vi "Get RT Driver Info - 331.vi"(8 "error in (no error)":errorcluster) -> (0 "error out":errorcluster, 1 "RT Driver Info":T1[](array[typedef]))   [LabVIEW 2018, in "FPGA Addon Shared.lvlib"]
uses:
  FPGA Addon Shared.lvlib
  <vilib>/NI/NI VeriStand Advanced SysDef API/_Types/Property.DependentFile.ctl
  NationalInstruments.VeriStand.SystemDefinitionAPI
  Constants.vi
  <vilib>/Utility/LVLibp/NI_PackedLibraryUtility.lvlib
  <vilib>/NI/NI VeriStand Advanced SysDef API/SysDef API/Advanced System Definition.lvlib
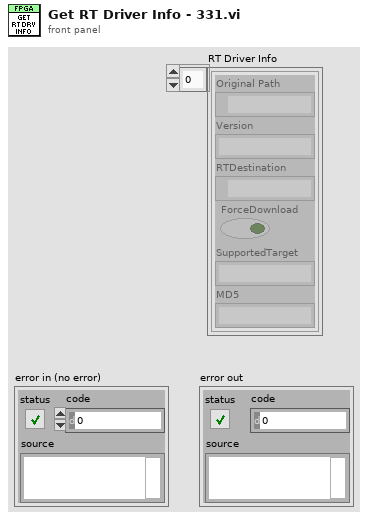
[diagram p1: front panel]
types:
  T1 = typedef "Advanced System Definition.lvlib/Property.DependentFile.ctl" = cluster{"Original Path":path, "Version":string, "RTDestination":path, "ForceDownload":bool, "SupportedTarget":string, "MD5":string}
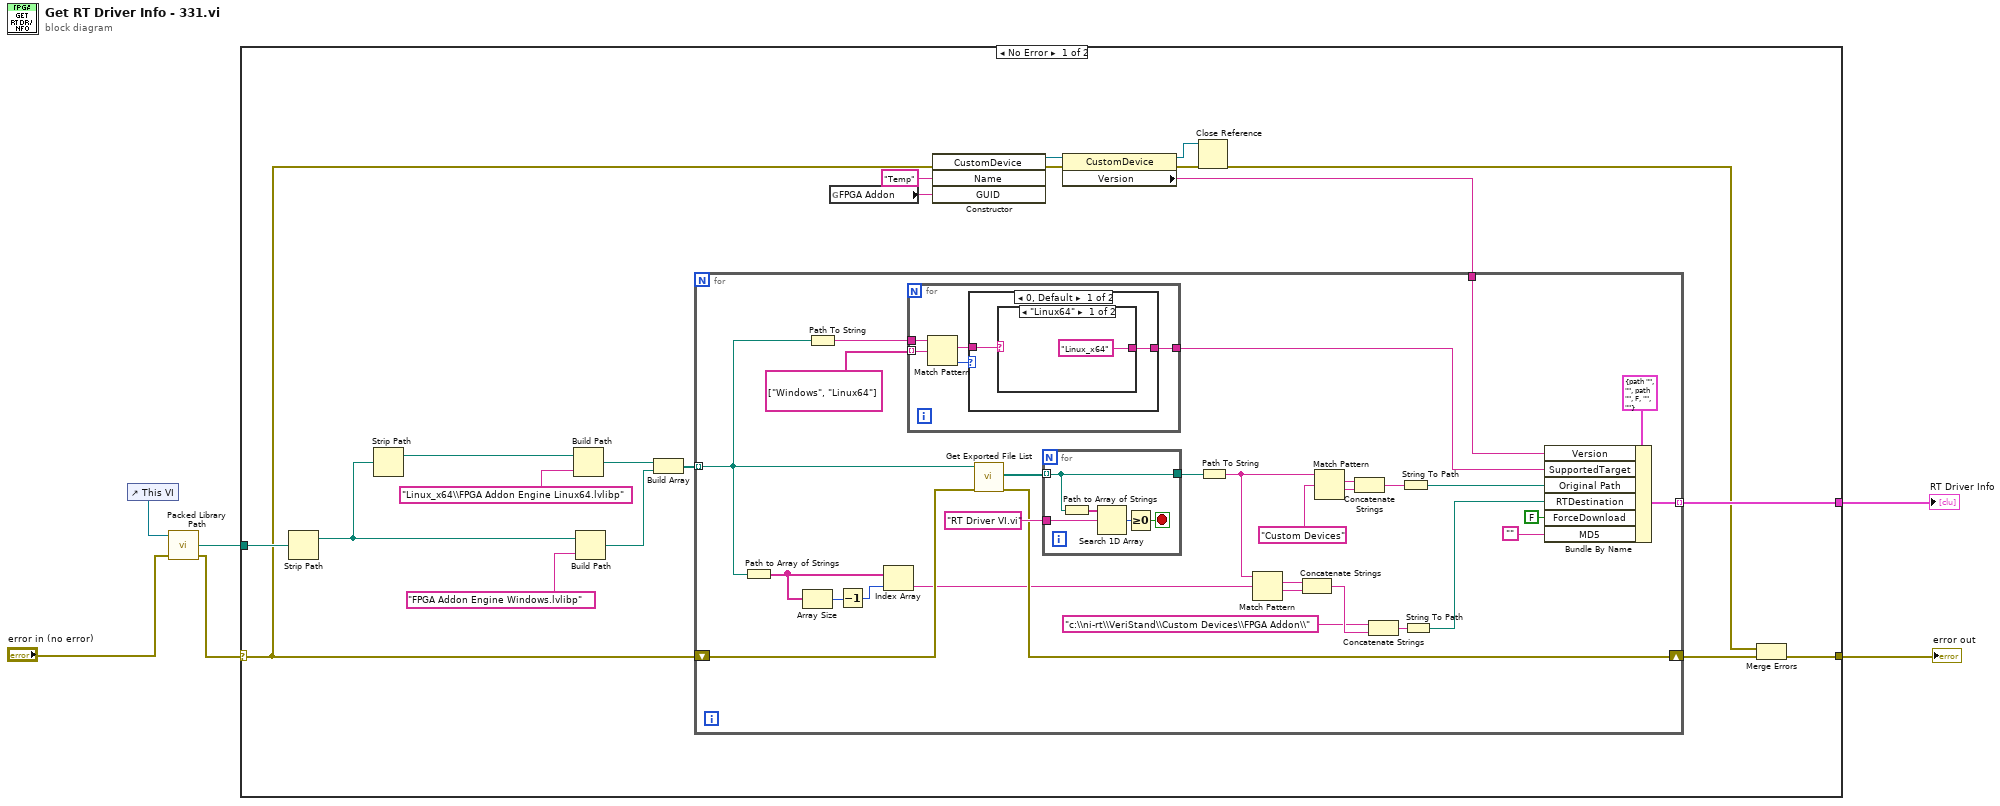
[diagram p0: block diagram]
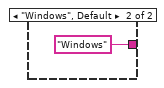
[diagram p2: hidden frame]
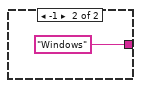
[diagram p3: hidden frame]
diagram:
  n1 = control-ref of="This VI"() -> (w3:refnum<vi>)
  n2 = call <vilib>:"Packed Library Path.vi"("error in (no error)"="error in (no error)", "vi reference"=w3) -> ("error out"=w2:errorcluster, "packed library path"=w6:path)  [unwired: 1 in, 1 out]
  n3 = case shown="No Error" w2 {
    selector: w2 -> [w10 w72]
    tunnel: w6 -> [w19 _]
    tunnel: [w7 w72] -> w4
    tunnel: [w18 _] -> w1
    frame No Error {
      n4 = Strip Path(path=w19) -> (stripped path=w23:path)  [unwired: 1 out]
      n5 = Strip Path(path=w23) -> (stripped path=w20:path)  [unwired: 1 out]
      n6 = Build Path(base path=w20, name or relative path="Linux_x64\\FPGA Addon Engine Linux64.lvlibp") -> (appended path=w24:path)
      n7 = Build Path(base path=w23, name or relative path="FPGA Addon Engine Windows.lvlibp") -> (appended path=w25:path)
      n8 = Build Array(w24, w25) -> (w26:path[])
      n9 = global read "Constants.vi" "FPGA Addon"() -> (w12:string)
      n10 = constructor class="CustomDevice"(error in=w10, "Name"="Temp", "GUID"=w12) -> (reference out=w17:refnum<k24>, error out=w16:errorcluster)  [unwired: 2 in, 3 out]
      n11 = property class="CustomDevice"(reference=w17, error in=w16) -> (reference out=w14:refnum<k24>, error out=w15:errorcluster, "Version"=w11:string)
      n12 = for {
        shift-right: [w53] -> w9
        shift-left: w10 -> [w54]
        tunnel: w26 -> [w33] mode=indexing
        tunnel: [w28] -> w18 mode=indexing
        tunnel: w11 -> [w27]
        n13 = Path to Array of Strings(0:w33) -> (2:w41:string[])  [unwired: 1 out]
        n14 = Array Size(array=w41) -> (size(s)=w43:i32)
        n15 = Path To String(path=w33) -> (string=w32:string)
        n16 = Decrement(x=w43) -> (x-1=w42:i32)
        n17 = Index Array(array=w41, index=w42) -> (element=w40:string)
        n18 = for {
          tunnel: w32 -> [w61]
          tunnel: string[] ["Windows", "Linux64"] -> [w60] mode=indexing
          tunnel: [w57] -> w30
          n19 = Match Pattern(string=w61, regular expression=w60) -> (match substring=w58:string, offset past match=w59:i32)  [unwired: 1 in, 2 out]
          n20 = case shown="0, Default" w59 {
            tunnel: w58 -> [w63 _]
            tunnel: [w62 "Windows" ("regular expression")] -> w57
            frame 0, Default {
              n21 = case shown="\"Linux64\"" w63 {
                tunnel: ["Linux_x64" ("regular expression") "Windows" ("regular expression")] -> w62
                frame "Linux64" {
                }
                frame "Windows", Default {
                }
              }
            }
            frame -1 {
            }
          }
        }
        n22 = call <vilib>:"Get Exported File List.vi"("error in (no error)"=w54, "packed library path"=w33) -> ("error out"=w53:errorcluster, "paths"=w56:path[])  [unwired: 7 in, 1 out]
        n23 = for {
          tunnel: w56 -> [w68] mode=indexing
          tunnel: "RT Driver VI.vi" ("element") -> [w70]
          tunnel: [w68] -> w52
          stop <- w67 stop-if-true
          n24 = Path to Array of Strings(0:w68) -> (2:w71:string[])  [unwired: 1 out]
          n25 = Search 1D Array(1D array=w71, element=w70) -> (index of element=w69:i32)  [unwired: 1 in]
          n26 = Greater Or Equal To 0?(x=w69) -> (x >= 0?=w67:bool)
        }
        n27 = Path To String(path=w52) -> (string=w48:string)
        n28 = Match Pattern(string=w48, regular expression=w40) -> (match substring=w47:string, after substring=w46:string)  [unwired: 1 in, 2 out]
        n29 = Concatenate Strings(w47, w46) -> (w45:string)
        n30 = Match Pattern(string=w48, regular expression="Custom Devices") -> (match substring=w50:string, after substring=w49:string)  [unwired: 1 in, 2 out]
        n31 = Concatenate Strings(w50, w49) -> (w38:string)
        n32 = Concatenate Strings("c:\\ni-rt\\VeriStand\\Custom Devices\\FPGA Addon\\" ("regular expression"), w45) -> (w36:string)
        n33 = String To Path(string=w38) -> (path=w37:path)
        n34 = String To Path(string=w36) -> (path=w35:path)
        n35 = Bundle By Name(cluster=T1 {"Original Path"=path "", "Version"="", "RTDestination"=path "", "ForceDownload"=FALSE, "SupportedTarget"="", "MD5"=""} ("OptionalInfo"), "Version"=w27, "SupportedTarget"=w30, "Original Path"=w37, "RTDestination"=w35, "ForceDownload"=FALSE, "MD5"="") -> (w28:T1)
      }
      n36 = Close Reference(reference=w14, error in (no error)=w15) -> (error out=w8:errorcluster)
      n37 = Merge Errors(w8, w9) -> (w7:errorcluster)
    }
    frame Error {
    }
  }
  "error out" <- w4
  "RT Driver Info" <- w1
